vi "Test Dog Bark.vi"(8 "error in (no error)":errorcluster, 11 "Dog Test In":refnum<class "Dog Test.lvclass">) -> (0 "error out":errorcluster, 3 "Dog Test Out":refnum<class "Dog Test.lvclass">)   [LabVIEW 2020, in "Dog Test.lvclass"]
doc: "Test Dog bark"
uses:
  Dog Test.lvclass
  C:/git/astemes-lunit/source/API/LUnit Test Case/LUnit Test Case.lvclass
  API/LUnit Test Case/LUnit Test Case.lvclass/LUnit Test Case.ctl
  3de7b966-a5ef-46c3-a354-cc7dc217bc5a.vi
  API/LUnit Test Case/Private/Append Pass Result.vi
  API/LUnit Test Case/Private/Append Fail Result.vi
  API/LUnit Test Case/Private/Compare Variants.vi
  API/LUnit Test Case/Private/Describe Comparison.vi
  API/LUnit Test Case/Private/Variant to string.vi
  <vilib>/Utility/Data Type/Get Type Information.vi
  <vilib>/Utility/LVClass/Get LV Class Name.vi
  Animal Classes/Dog/Dog.lvclass
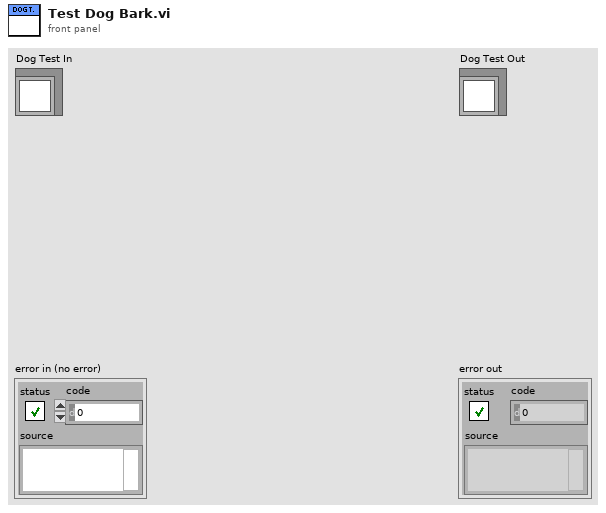
[diagram p1: front panel]
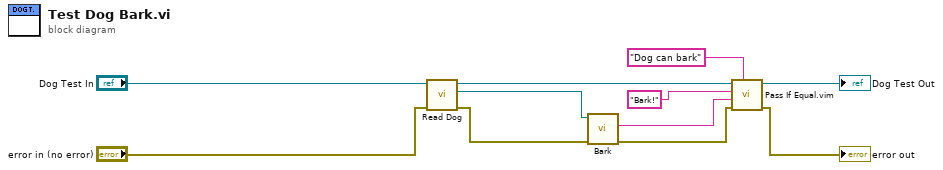
[diagram p0: block diagram]
diagram:
  n1 = call "Read Dog.vi"("error in (no error)"="error in (no error)", "Dog Test in"="Dog Test In") -> ("error out"=w8:errorcluster, "Dog.lvclass"=w9:refnum<class "Dog.lvclass">, "Dog Test out"=w7:refnum<class "Dog Test.lvclass">)  [unwired: 7 in]
  n2 = call "Bark.vi"("error in (no error)"=w8, "Dog In"=w9) -> ("error out"=w2:errorcluster, "Result"=w4:string)  [unwired: 7 in, 1 out]
  n3 = call "Pass If Equal.vim"("Description"="Dog can bark", "error in (no error)"=w2, "Actual"=w4, "Expected"="Bark!", "LUnit Test Case In"=w7) -> ("error out"=→"error out":errorcluster, "LUnit Test Case Out"=→"Dog Test Out":refnum<class "Dog Test.lvclass">)  [unwired: 5 in]
